vi "AudioTest.SoundCheck Data Log Graph Window - Single.vi"() -> ()   [LabVIEW 2018]
uses:
  TypeDefs/AudioTest.Analysis Data Record.ctl
  <vilib>/Utility/miscctls.llb/LVRectTypeDef.ctl
  <vilib>/KATE/Queues/Queue Utils.lvlib
  <vilib>/KATE/Files/File Utils.lvlib
  <vilib>/KATE/Controls/Controls.lvlib
panel:
  in  "Main Tab":enum32{"Data", "Setup"}(tab)
  out "Fail":bool
  out "Graph1 1":cluster{"X":dbl[], "Y":dbl[]}[](graph)
  in  "Graph":T1
  in  "Config Folder":path=path "C:/MTE/Audio Test/Config"
  in  "QName":string="Plot_00"
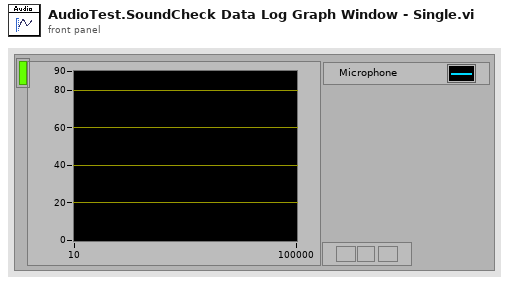
[diagram p1: front panel]
types:
  T1 = typedef "AudioTest.Analysis Data Record.ctl" = cluster{"Name":string, "X Units":string, "Y Units":string, "DataPlots":cluster{"X":dbl[], "Y":dbl[]}[], "LimitPlots":cluster{"X":dbl[], "Y":dbl[]}[], "DataPlotNames":string[], "LimitPlotNames":string[], "Fail":bool}
  T2 = enum32{"Invalid", "Standard", "Closed", "Hidden", "Minimized", "Maximized"}
  T3 = typedef "LVRectTypeDef.ctl" = cluster{"Left":i16, "Top":i16, "Right":i16, "Bottom":i16}
  T4 = enum16{"Top Left", "Bottom Right", "Top Right", "Bottom Left"}
  T5 = cluster{"Graphs":T1[], "PlotColors":u32[], "LimColors":u32[]}
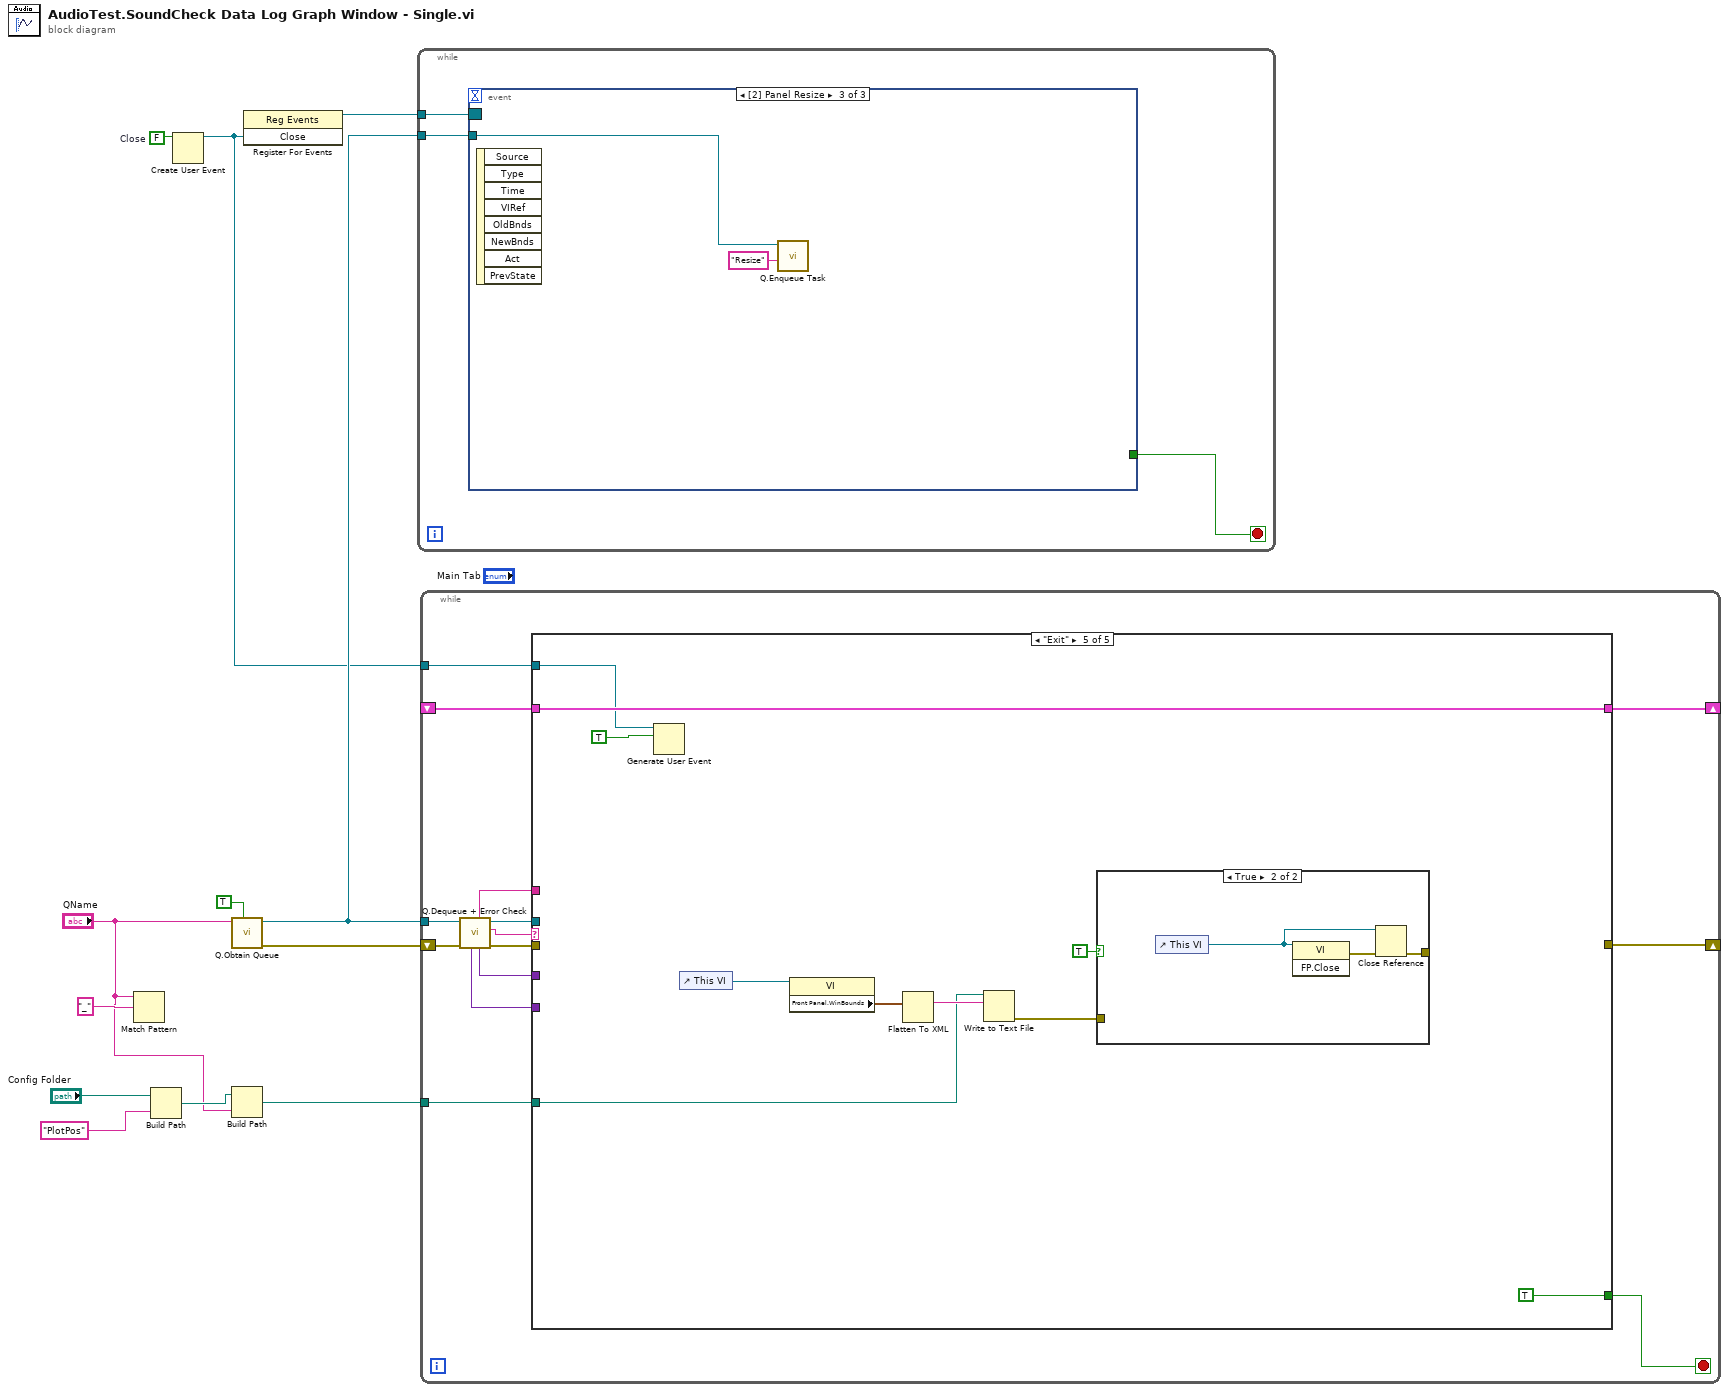
[diagram p0: block diagram]
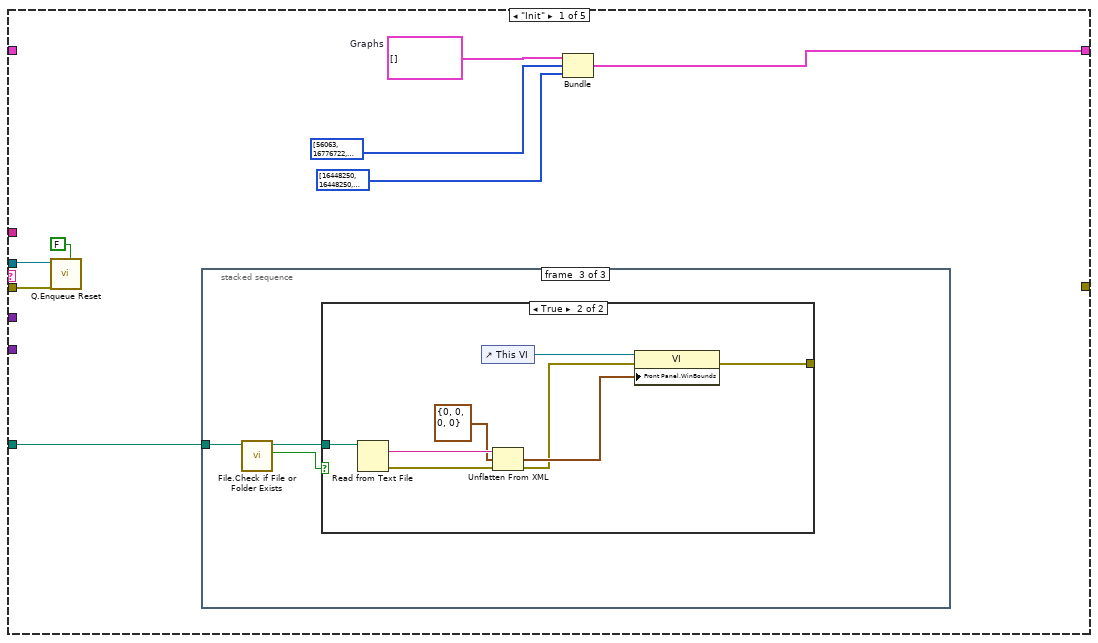
[diagram p2: hidden frame]
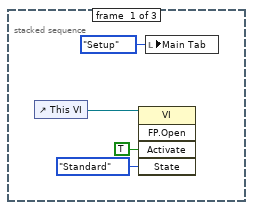
[diagram p3: hidden frame]
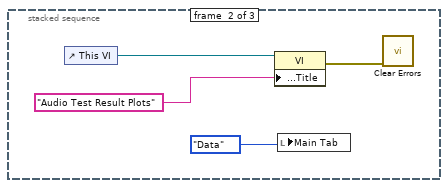
[diagram p4: hidden frame]
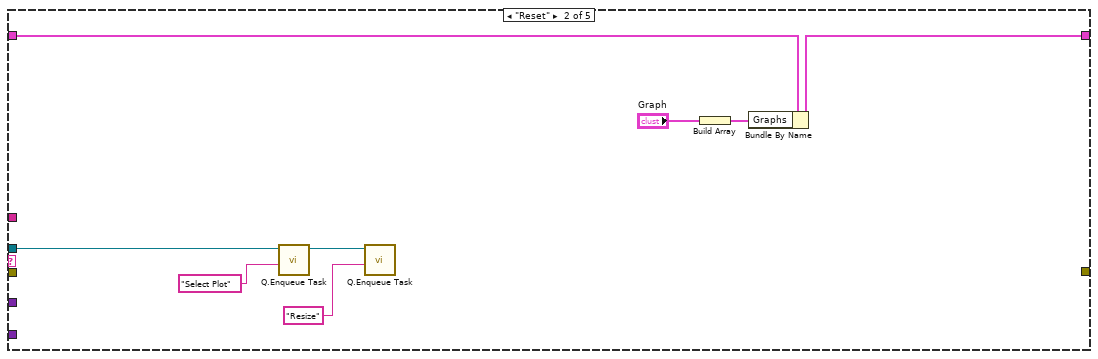
[diagram p6: hidden frame]
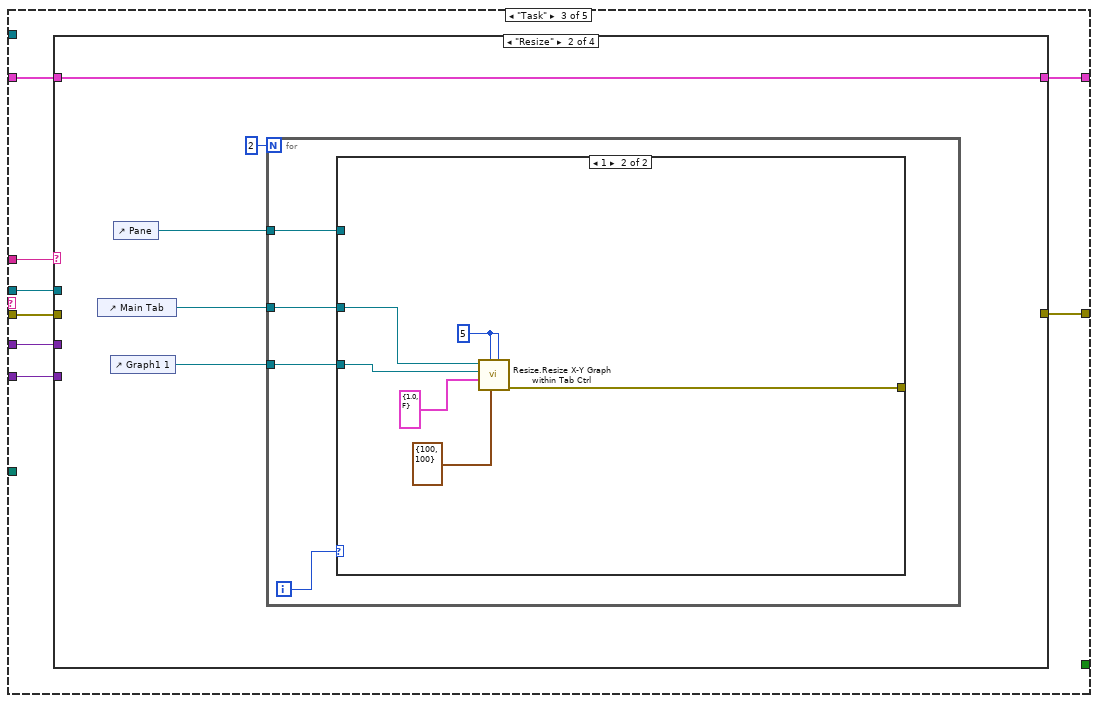
[diagram p7: hidden frame]
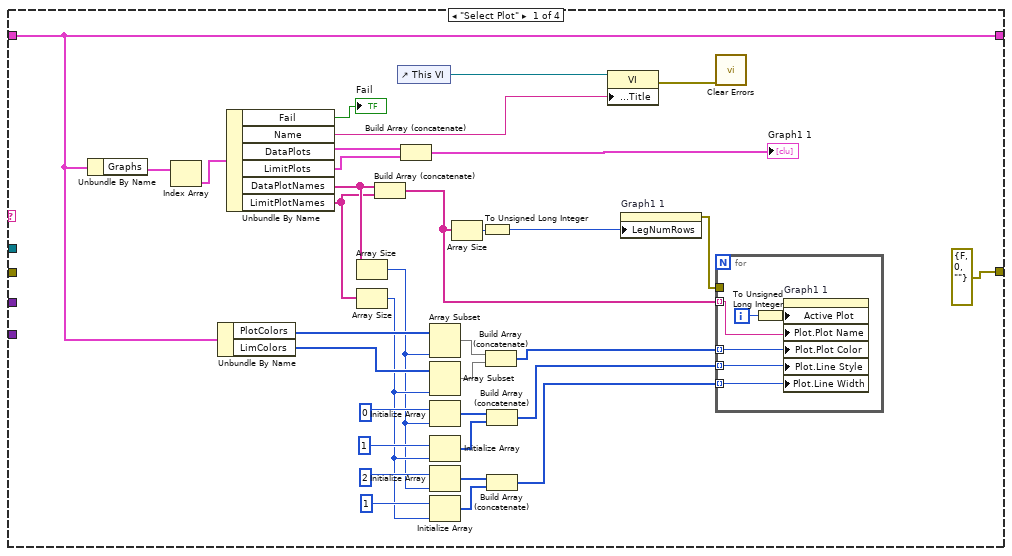
[diagram p8: hidden frame]
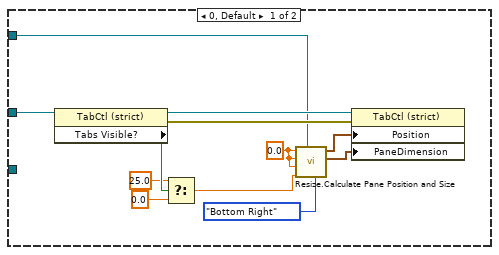
[diagram p9: hidden frame]
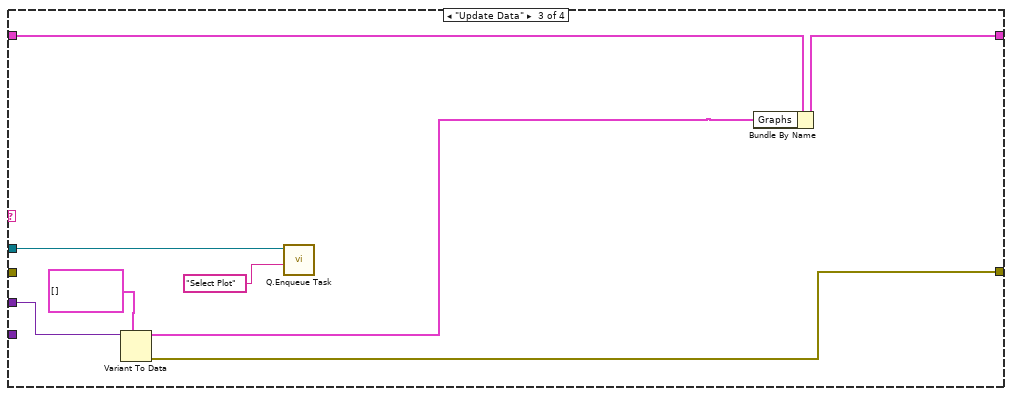
[diagram p10: hidden frame]
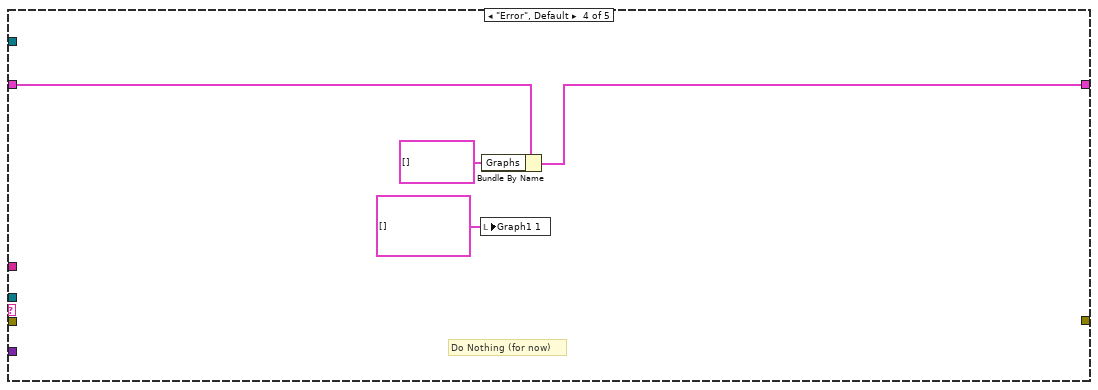
[diagram p12: hidden frame]
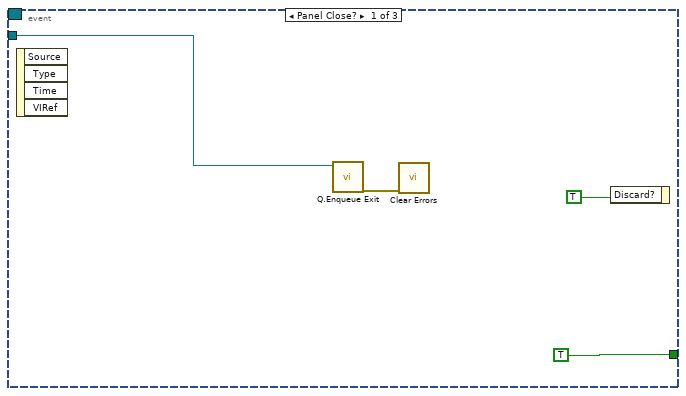
[diagram p14: hidden frame]
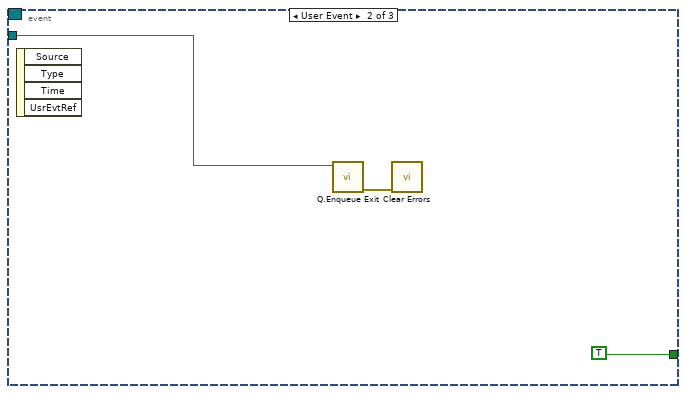
[diagram p15: hidden frame]
diagram:
  w12 = FALSE  # Close
  n1 = Match Pattern(string="QName", regular expression="_") -> ()  [unwired: 1 in, 4 out]
  n2 = Build Path(base path="Config Folder", name or relative path="PlotPos" ("regular expression")) -> (appended path=w3:path)
  n3 = Create User Event(user event datatype=w12) -> (user event=w7:refnum<user-event>)  [unwired: 1 in, 1 out]
  n4 = call <vilib>:"Q.Obtain Queue.vi"("Enqueue Init"=TRUE, "Q Name"="QName") -> ("error out"=w9:errorcluster, "Q Out"=w8:refnum<queue>)  [unwired: 7 in, 1 out]
  n5 = Build Path(base path=w3, name or relative path="QName") -> (appended path=w1:path)
  n6 = register-events(w7) -> (reference out=w11:refnum<event-registration>)  [unwired: 2 in, 1 out]
  n7 = while {
    tunnel: w11 -> [w15]
    tunnel: w8 -> [w14]
    stop <- w13 stop-if-true
    n8 = event shown="[2] Panel Resize" {
      selector: w15 -> [_ _ _]
      dyn-events: _ -> [_ _ _]
      timeout: _ -> [_ _ _]
      tunnel: w14 -> [w18 w21 w24]
      tunnel: [TRUE TRUE _] -> w13
      event Panel Close? {
        n9 = event-data() -> ()  [unwired: 1 in, 4 out]
        n10 = call <vilib>:"Q.Enqueue Exit.vi"("Q In"=w18) -> ("error out"=w17:errorcluster)  [unwired: 9 in, 1 out]
        n11 = call <vilib>:"Clear Errors.vi"("error in (no error)"=w17) -> ()  [unwired: 5 in, 2 out]
        n12 = event-data("Discard?"=TRUE) -> ()  [unwired: 1 in, 1 out]
      }
      event User Event {
        n13 = event-data() -> ()  [unwired: 1 in, 4 out]
        n14 = call <vilib>:"Q.Enqueue Exit.vi"("Q In"=w21) -> ("error out"=w20:errorcluster)  [unwired: 9 in, 1 out]
        n15 = call <vilib>:"Clear Errors.vi"("error in (no error)"=w20) -> ()  [unwired: 5 in, 2 out]
      }
      event Panel Resize {
        n16 = event-data() -> ()  [unwired: 1 in, 8 out]
        n17 = call <vilib>:"Q.Enqueue Task.vi"("Task Name"="Resize", "Q In"=w24) -> ()  [unwired: 8 in, 2 out]
      }
    }
  }
  n18 = while {
    shift-right: [w30] -> _
    shift-left: w9 -> [w35]
    tunnel: w8 -> [w33]
    shift-right: [w28] -> _
    shift-left: _ -> [w27]
    tunnel: w7 -> [w26]
    tunnel: w1 -> [w25]
    stop <- w29 stop-if-true
    n19 = call <vilib>:"Q.Dequeue + Error Check.vi"("Error In"=w35, "Q In"=w33) -> ("error out"=w36:errorcluster, "Cmd"=w38:string, "Q Out"=w37:refnum<queue>, "Data1"=w32:variant, "Sub"=w34:string, "Data2"=w31:variant)  [unwired: 4 in]
    n20 = case shown="\"Exit\"" w38 {
      tunnel: w37 -> [w46 w71 w80 _ _]
      tunnel: w36 -> [w45 _ w79 _ _]
      tunnel: w34 -> [_ _ w81 _ _]
      tunnel: w32 -> [_ _ w78 _ _]
      tunnel: w31 -> [_ _ w77 _ _]
      tunnel: [_ _ w74 _ _] -> w30
      tunnel: [_ _ _ _ TRUE] -> w29
      tunnel: [w40 w73 w75 w160 w170] -> w28
      tunnel: w27 -> [_ w72 w76 w161 w170]
      tunnel: w26 -> [_ _ _ _ w169]
      tunnel: w25 -> [w39 _ _ _ w163]
      frame "Init" {
        w43 = T1[] []  # Graphs
        n21 = call <vilib>:"Q.Enqueue Reset.vi"("Top of Q(T)"=FALSE, "Error In"=w45, "Q In"=w46) -> ()  [unwired: 7 in, 2 out]
        n22 = stacked-sequence {
          tunnel: w39 -> [_ _ w57]
          frame #0 {
            n23 = control-ref of="This VI"() -> (w50:refnum<vi>)
            n24 = invoke class="VI" method="FP.Open"(reference=w50, "Activate"=TRUE ("Activate?"), "State"=T2."Standard") -> ()  [unwired: 2 in, 5 out]
            n25 = local write "Main Tab"(enum32{"Data", "Setup"}."Setup" ("Main Tab")) -> ()
          }
          frame #1 {
            n26 = control-ref of="This VI"() -> (w54:refnum<vi>)
            n27 = property class="VI"(reference=w54, "Front Panel.Title"="Audio Test Result Plots") -> (error out=w53:errorcluster)  [unwired: 1 in, 1 out]
            n28 = local write "Main Tab"(enum32{"Data", "Setup"}."Data" ("Main Tab")) -> ()
            n29 = call <vilib>:"Clear Errors.vi"("error in (no error)"=w53) -> ()  [unwired: 5 in, 2 out]
          }
          frame #2 {
            n30 = call <vilib>:"File.Check if File or Folder Exists.vi"("Path"=w57) -> ("Exists"=w55:bool, "Dup Path"=w56:path)  [unwired: 6 in, 3 out]
            n31 = case shown="True" w55 {
              tunnel: w56 -> [_ w64]
              tunnel: [_ w58] -> _
              frame False {
              }
              frame True {
                n32 = Read from Text File(file (use dialog)=w64) -> (text=w63:string, error out=w59:errorcluster)  [unwired: 3 in, 2 out]
                n33 = control-ref of="This VI"() -> (w65:refnum<vi>)
                n34 = Unflatten From XML(xml string=w63, type=T3 {"Left"=0, "Top"=0, "Right"=0, "Bottom"=0} ("Front Panel Window:Window Bounds"), error in (no error)=w59) -> (value=w61:T3, error out=w60:errorcluster)
                n35 = property class="VI"(reference=w65, error in=w60, "Front Panel.WinBounds"=w61) -> (error out=w58:errorcluster)  [unwired: 1 out]
              }
            }
          }
        }
        n36 = Bundle("Graphs"=w43, "PlotColors"=u32[] [56063, 16776722, 16730898, 16711925, 6618880], "LimColors"=u32[] [16448250, 16448250, 16448250, 16448250, 16448250, 16448250]) -> (w40:T5)  [unwired: 1 in]
      }
      frame "Reset" {
        n37 = call <vilib>:"Q.Enqueue Task.vi"("Task Name"="Select Plot", "Q In"=w71) -> ("Q Out"=w68:refnum<queue>)  [unwired: 8 in, 1 out]
        n38 = call <vilib>:"Q.Enqueue Task.vi"("Task Name"="Resize", "Q In"=w68) -> ()  [unwired: 8 in, 2 out]
        n39 = Build Array("Graph") -> (w67:T1[])
        n40 = Bundle By Name(cluster=w72, "Graphs"=w67) -> (w73:T5)
      }
      frame "Task" {
        n41 = case shown="\"Resize\"" w81 {
          tunnel: w80 -> [_ _ w155 _]
          tunnel: w79 -> [_ _ _ _]
          tunnel: w78 -> [_ _ w152 _]
          tunnel: w77 -> [_ _ _ _]
          tunnel: w76 -> [w115 w126 w154 w157]
          tunnel: [w115 w126 w153 w157] -> w75
          tunnel: [errorcluster {"status"=FALSE, "code"=0, "source"=""} ("error constant") _ w151 _] -> w74
          frame "Select Plot" {
            n42 = Unbundle By Name(w115) -> ("Graphs"=w87:T1[])
            n43 = Index Array(array=w87) -> (element=w86:T1)  [unwired: 1 in]
            n44 = Unbundle By Name(w115) -> ("PlotColors"=w106:u32[], "LimColors"=w105:u32[])
            n45 = Unbundle By Name(w86) -> ("Fail"=→"Fail":bool, "Name"=w83:string, "DataPlots"=w113:cluster{"X":dbl[], "Y":dbl[]}[], "LimitPlots"=w112:cluster{"X":dbl[], "Y":dbl[]}[], "DataPlotNames"=w108:string[], "LimitPlotNames"=w107:string[])
            n46 = Array Size(array=w108) -> (size(s)=w91:i32)
            n47 = Array Size(array=w107) -> (size(s)=w92:i32)
            n48 = Build Array (concatenate)(w108, w107) -> (w109:string[])
            n49 = control-ref of="This VI"() -> (w85:refnum<vi>)
            n50 = Build Array (concatenate)(w113, w112) -> (→"Graph1 1":cluster{"X":dbl[], "Y":dbl[]}[])
            n51 = Array Subset(array=w106, length=w91) -> (w104:u32[])  [unwired: 1 in]
            n52 = Array Subset(array=w105, length=w92) -> (w103:u32[])  [unwired: 1 in]
            n53 = Initialize Array(u8 0 ("Plot.Line Style"), w91) -> (w99:u8[])
            n54 = Initialize Array(u8 1 ("Plot.Line Style"), w92) -> (w98:u8[])
            n55 = Initialize Array(u8 2 ("Plot.Line Style"), w91) -> (w95:u8[])
            n56 = Initialize Array(u8 1 ("Plot.Line Style"), w92) -> (w96:u8[])
            n57 = Array Size(array=w109) -> (size(s)=w111:i32)
            n58 = To Unsigned Long Integer(number=w111) -> (unsigned 32bit integer=w110:u32)
            n59 = Build Array (concatenate)(w104, w103) -> (w102:u32[])
            n60 = Build Array (concatenate)(w99, w98) -> (w97:u8[])
            n61 = Build Array (concatenate)(w95, w96) -> (w90:u8[])
            n62 = property class="VI"(reference=w85, "Front Panel.Title"=w83) -> (error out=w84:errorcluster)  [unwired: 1 in, 1 out]
            n63 = property on="Graph1 1" class="XYGraph (strict)"("LegNumRows"=w110) -> (error out=w88:errorcluster)  [unwired: 2 in, 1 out]
            n64 = call <vilib>:"Clear Errors.vi"("error in (no error)"=w84) -> ()  [unwired: 5 in, 2 out]
            n65 = for {
              tunnel: w109 -> [w119] mode=indexing
              tunnel: w88 -> [_]
              tunnel: w102 -> [w118] mode=indexing
              tunnel: w97 -> [w117] mode=indexing
              tunnel: w90 -> [w116] mode=indexing
              i -> [w120]
              n66 = To Unsigned Long Integer(number=w120) -> (unsigned 32bit integer=w121:u32)
              n67 = property on="Graph1 1" class="XYGraph (strict)"("Active Plot"=w121, "Plot.Plot Name"=w119, "Plot.Plot Color"=w118, "Plot.Line Style"=w117, "Plot.Line Width"=w116) -> ()  [unwired: 2 in, 2 out]
            }
          }
          frame "Resize" {
            n68 = control-ref of="Main Tab"() -> (w125:refnum<vi>)
            n69 = control-ref of="Graph1 1"() -> (w124:refnum<vi>)
            n70 = control-ref of="Pane"() -> (w123:refnum<vi>)
            n71 = for {
              N: 2 -> [_]
              tunnel: w125 -> [w129]
              tunnel: w124 -> [w128]
              tunnel: w123 -> [w127]
              i -> [w130]
              n72 = case shown="1" w130 {
                tunnel: w129 -> [w132 w148]
                tunnel: w128 -> [_ w147]
                tunnel: w127 -> [w131 _]
                tunnel: [_ w143] -> _
                frame 0, Default {
                  w135 = 0.0 ("X Origin")
                  n73 = property class="TabCtl (strict)"(reference=w132) -> (reference out=w142:refnum<vi>, error out=w138:errorcluster, "Tabs Visible?"=w141:bool)  [unwired: 1 in]
                  n74 = Select(t=25.0, s=w141, f=0.0) -> (s? t:f=w134:dbl)
                  n75 = call <vilib>:"Resize.Calculate Pane Position and Size.vi"("Origin for X,Y Max (Top Left)"=T4."Bottom Right", "Pane in"=w131, "Y Max"=w134, "X Max"=w135, "Y Origin"=w135, "X Origin"=w135) -> ("Size"=w136:cluster{u32, u32}, "Position"=w137:cluster{"X Coordinate":i32, "Y Coordinate":i32})  [unwired: 4 in]
                  n76 = property class="TabCtl (strict)"(reference=w142, error in=w138, "Position"=w137, "PaneDimension"=w136) -> ()  [unwired: 2 out]
                }
                frame 1 {
                  w144 = 5 ("Pix from Right")
                  n77 = call <vilib>:"Resize.Resize X-Y Graph within Tab Ctrl.vi"("Pix from Bottom"=w144, "Min Size"=cluster{"Width":i32, "Height":i32} {"Width"=100, "Height"=100}, "Pix from Right"=w144, "Aspect Ratio"=cluster{"W/H":dbl, "Enable":bool} {"W/H"=1.0, "Enable"=FALSE}, "X-Y Graph Ctrl"=w147, "Tab Ctrl"=w148) -> ("error out"=w143:errorcluster)  [unwired: 3 in, 2 out]
                }
              }
            }
          }
          frame "Update Data" {
            n78 = Variant To Data(type=T1[] [] ("Graphs"), Variant=w152) -> (data=w150:T1[], error out=w151:errorcluster)  [unwired: 1 in]
            n79 = call <vilib>:"Q.Enqueue Task.vi"("Task Name"="Select Plot", "Q In"=w155) -> ()  [unwired: 8 in, 2 out]
            n80 = Bundle By Name(cluster=w154, "Graphs"=w150) -> (w153:T5)
          }
          frame Default {
          }
        }
      }
      frame "Error", Default {
        # "Do Nothing (for now)"
        n81 = local write "Graph1 1"(cluster{"X":dbl[], "Y":dbl[]}[] [] ("XY Graph")) -> ()
        n82 = Bundle By Name(cluster=w161, "Graphs"=T1[] []) -> (w160:T5)
      }
      frame "Exit" {
        n83 = Generate User Event(user event=w169, event data cluster=TRUE ("event data")) -> ()  [unwired: 2 in, 2 out]
        n84 = control-ref of="This VI"() -> (w166:refnum<vi>)
        n85 = property class="VI"(reference=w166) -> ("Front Panel.WinBounds"=w165:T3)  [unwired: 1 in, 2 out]
        n86 = Flatten To XML(anything=w165) -> (xml string=w164:string)
        n87 = Write to Text File(file (use dialog)=w163, text=w164) -> (error out=w162:errorcluster)  [unwired: 2 in, 2 out]
        n88 = case shown="True" TRUE {
          tunnel: [_ w172] -> _
          tunnel: w162 -> [_ _]
          frame False {
          }
          frame True {
            n89 = control-ref of="This VI"() -> (w174:refnum<vi>)
            n90 = invoke class="VI" method="FP.Close"(reference=w174) -> (error out=w173:errorcluster)  [unwired: 2 in, 2 out]
            n91 = Close Reference(reference=w174, error in (no error)=w173) -> (error out=w172:errorcluster)
          }
        }
      }
    }
  }
